vi "Preprocess.vi"(11 "Input(Targter/Nontarget_ERP)":dbl[][](array[numeric])) -> (1 "STD":dbl[](array[numeric]), 2 "Average":dbl[](array[numeric]), 3 "ouput":dbl[][](array[numeric]))   [LabVIEW 2013]
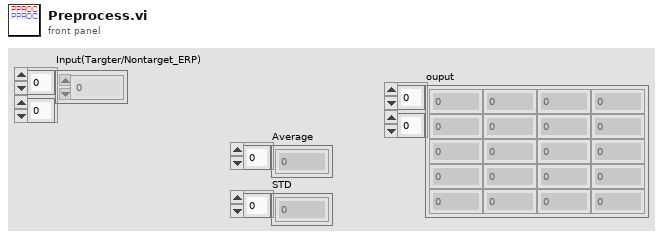
[diagram p1: front panel]
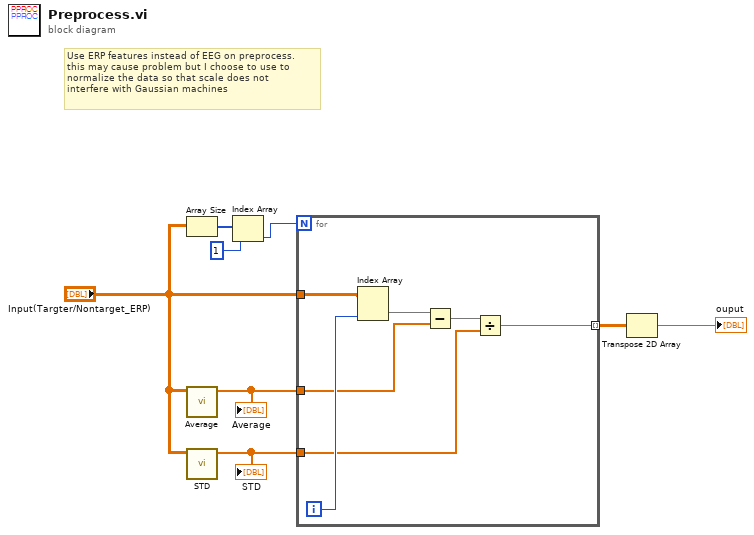
[diagram p0: block diagram]
diagram:
  # "Use ERP features instead of EEG on preprocess.\nthis may cause problem but I choose to use to\nnormalize the data so that scale does not \ninterfere with Gaussian machines"
  n1 = Array Size(array="Input(Targter/Nontarget_ERP)") -> (size(s)=w8:i32[])
  n2 = call "Average.vi"("Input_array"="Input(Targter/Nontarget_ERP)") -> ("Average"=w5:dbl[])  [unwired: 10 in]
  "Average" <- w5
  n3 = call "STD.vi"("Input_array"="Input(Targter/Nontarget_ERP)") -> ("STD"=w4:dbl[])  [unwired: 10 in]
  "STD" <- w4
  n4 = Index Array(array=w8, index=1) -> (element=w7:i32)
  n5 = for {
    N: w7 -> [_]
    tunnel: w5 -> [w12]
    tunnel: w4 -> [w11]
    tunnel: "Input(Targter/Nontarget_ERP)" -> [w15]
    tunnel: [w10] -> w2 mode=indexing
    i -> [w14]
    n6 = Index Array(array=w15, index (col)=w14) -> (element=w13:dbl[])  [unwired: 1 in]
    n7 = Subtract(x=w13, y=w12) -> (x-y=w9:dbl[])
    n8 = Divide(x=w9, y=w11) -> (x/y=w10:dbl[])
  }
  n9 = Transpose 2D Array(2D array=w2) -> (transposed array=→"ouput":dbl[][])
